vi "WriteXML.vi"(8 "error in (no error)":errorcluster, 10 "Path":path, 11 "PixelflySettings in":refnum<class "PixelflySettings.lvclass">) -> (0 "error out":errorcluster, 3 "PixelflySettings out":refnum<class "PixelflySettings.lvclass">)   [LabVIEW 2009, in "Tools.lvlib" / "Settings.lvlib" / "PixelflySettings.lvclass"]
uses:
  PixelflySettings.lvclass
  NativeXML/NativeXML.lvclass
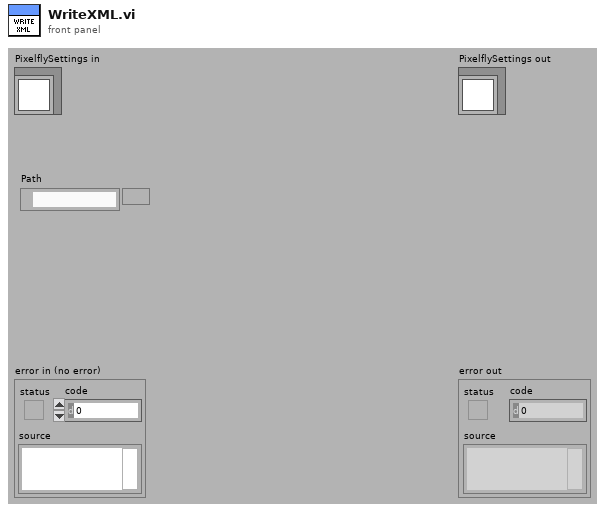
[diagram p1: front panel]
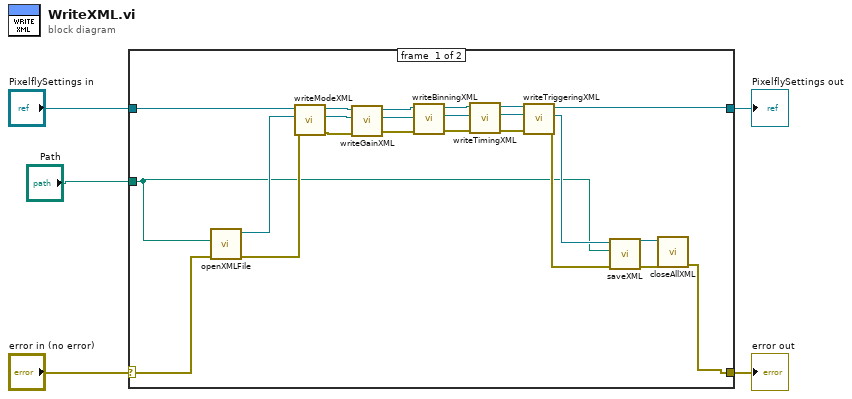
[diagram p0: block diagram]
diagram:
  n1 = case shown="No Error" "error in (no error)" {
    selector: "error in (no error)" -> [w12 w30]
    tunnel: [w6 w30] -> w4
    tunnel: [w23 w29] -> w2
    tunnel: "PixelflySettings in" -> [w28 w29]
    tunnel: "Path" -> [w9 _]
    frame #0 {
      n2 = call "openXMLFile.vi"("error in (no error)"=w12, "Path"=w9) -> ("error out"=w13:errorcluster, "NativeXML out"=w14:refnum<class "NativeXML.lvclass">)  [unwired: 8 in]
      n3 = call "writeModeXML.vi"("error in (no error)"=w13, "NativeXML in"=w14, "PixelflySettings in"=w28) -> ("error out"=w15:errorcluster, "NativeXML out"=w22:refnum<class "NativeXML.lvclass">, "PixelflySettings out"=w27:refnum<class "PixelflySettings.lvclass">)  [unwired: 6 in]
      n4 = call "writeGainXML.vi"("error in (no error)"=w15, "NativeXML in"=w22, "PixelflySettings in"=w27) -> ("error out"=w16:errorcluster, "NativeXML out"=w21:refnum<class "NativeXML.lvclass">, "PixelflySettings out"=w26:refnum<class "PixelflySettings.lvclass">)  [unwired: 6 in]
      n5 = call "writeBinningXML.vi"("error in (no error)"=w16, "NativeXML in"=w21, "PixelflySettings in"=w26) -> ("error out"=w17:errorcluster, "NativeXML out"=w20:refnum<class "NativeXML.lvclass">, "PixelflySettings out"=w25:refnum<class "PixelflySettings.lvclass">)  [unwired: 6 in]
      n6 = call "writeTimingXML.vi"("error in (no error)"=w17, "NativeXML in"=w20, "PixelflySettings in"=w25) -> ("error out"=w18:errorcluster, "NativeXML out"=w19:refnum<class "NativeXML.lvclass">, "PixelflySettings out"=w24:refnum<class "PixelflySettings.lvclass">)  [unwired: 6 in]
      n7 = call "writeTriggeringXML.vi"("error in (no error)"=w18, "NativeXML in"=w19, "PixelflySettings in"=w24) -> ("error out"=w10:errorcluster, "NativeXML out"=w11:refnum<class "NativeXML.lvclass">, "PixelflySettings out"=w23:refnum<class "PixelflySettings.lvclass">)  [unwired: 6 in]
      n8 = call "saveXML.vi"("error in (no error)"=w10, "Path"=w9, "NativeXML in"=w11) -> ("error out"=w8:errorcluster, "NativeXML out"=w7:refnum<class "NativeXML.lvclass">)  [unwired: 7 in]
      n9 = call "closeAllXML.vi"("error in (no error)"=w8, "NativeXML in"=w7) -> ("error out"=w6:errorcluster)  [unwired: 9 in]
    }
    frame #1 {
    }
  }
  "error out" <- w4
  "PixelflySettings out" <- w2
